vi "Event Handler.vi"(8 "error in (no error)":errorcluster, 10 "Stop Event Handler":refnum<user-event>, 11 "XYGraphOverview in":refnum<class "XYGraphOverview.lvclass">) -> (0 "error out":errorcluster)   [LabVIEW 2020, in "XYGraphOverview.lvlib" / "XYGraphOverview.lvclass"]
doc: "The <b>Event Handler VI</b> is a dynamic dispatch VI that should be overwritten if events are needed to create the enhanced QControl. \n\nBy inheriting from the main Control.lvclass the overwritten <b>Event Handler VI</b> will be launched asynchronously in the initialization of the QControl.\n<b> </b> <b> </b>\n©2016 Q Software Innovations, LLC (QSI)\nwritten by Quentin Alldredge\nproduced in LabVIEW 2015\n\nsupport@qsoftwareinnovations.com\nwww.qsoftwareinnovations.com\n\nAll rights reserved.\n\nRedistribution and use in source and binary forms, with or without modification, are permitted provided that the following conditions are met:\n\n * Redistributions of source code must retain the above copyright notice, this list of conditions and the following disclaimer.\n * Redistributions in binary form must reproduce the above copyright notice, this list of conditions and the following disclaimer in the documentation and/or other materials provided with the distribution.\n * Neither the name of Q Software Innovations, LLC. nor the names of its contributors may be used to endorse or promote products derived from this software without specific prior written permission.\n\nTHIS SOFTWARE IS PROVIDED BY THE COPYRIGHT HOLDERS AND CONTRIBUTORS \"AS IS\" AND ANY EXPRESS OR IMPLIED WARRANTIES, INCLUDING, BUT NOT LIMITED TO, THE IMPLIED WARRANTIES OF MERCHANTABILITY AND FITNESS FOR A PARTICULAR PURPOSE ARE DISCLAIMED. IN NO EVENT SHALL THE COPYRIGHT OWNER OR CONTRIBUTORS BE LIABLE FOR ANY DIRECT, INDIRECT, INCIDENTAL, SPECIAL, EXEMPLARY, OR CONSEQUENTIAL DAMAGES (INCLUDING, BUT NOT LIMITED TO, PROCUREMENT OF SUBSTITUTE GOODS OR SERVICES; LOSS OF USE, DATA, OR PROFITS; OR BUSINESS INTERRUPTION) HOWEVER CAUSED AND ON ANY THEORY OF LIABILITY, WHETHER IN CONTRACT, STRICT LIABILITY, OR TORT (INCLUDING NEGLIGENCE OR OTHERWISE) ARISING IN ANY WAY OUT OF THE USE OF THIS SOFTWARE, EVEN IF ADVISED OF THE POSSIBILITY OF SUCH DAMAGE."
uses:
  XYGraphOverview.lvclass
  XYGraphOverview.lvclass/XYGraphOverview.ctl
  X Range Change User Event Data.ctl
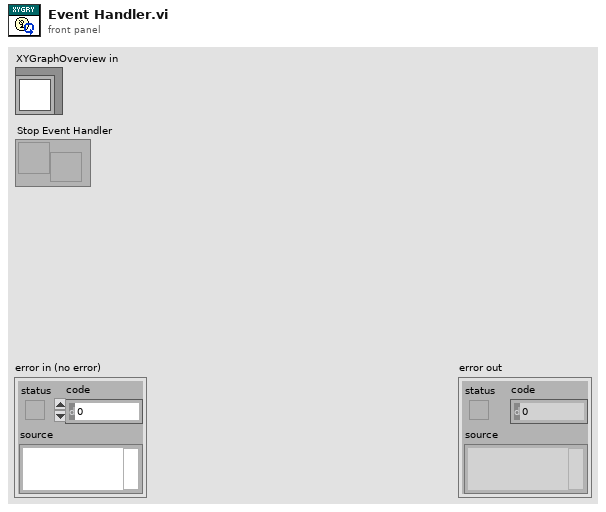
[diagram p1: front panel]
types:
  T1 = typedef "XYGraphOverview.lvlib/XYGraphOverview.lvclass/X Range Change User Event Data.ctl" = cluster{"Lower Range":dbl, "Upper Range":dbl, "All":bool}
  T2 = typedef "XYGraphOverview.lvlib/XYGraphOverview.lvclass/Command.ctl" = enum16{"Update Data", "Update Limit", "Zoom"}
  T3 = typedef "LVPoint32TypeDef.ctl" = cluster{"Horizontal":i32, "Vertical":i32}
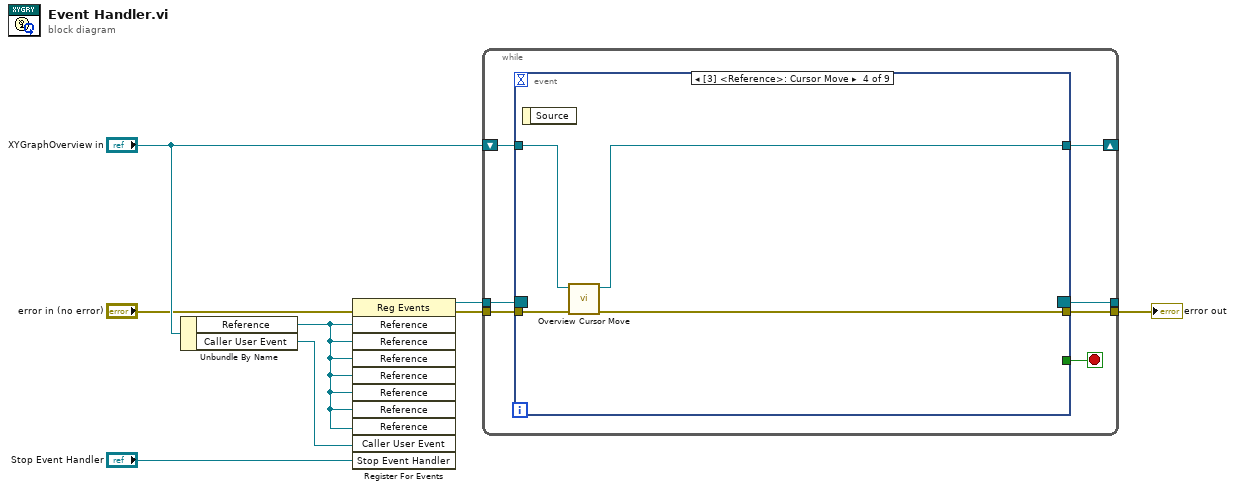
[diagram p0: block diagram]
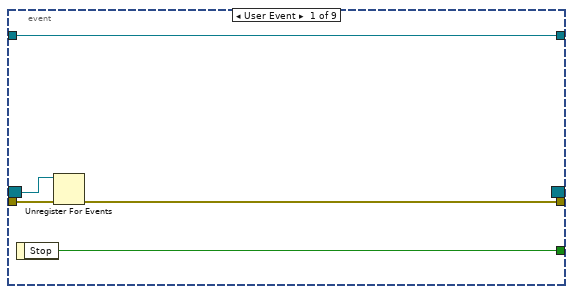
[diagram p2: hidden frame]
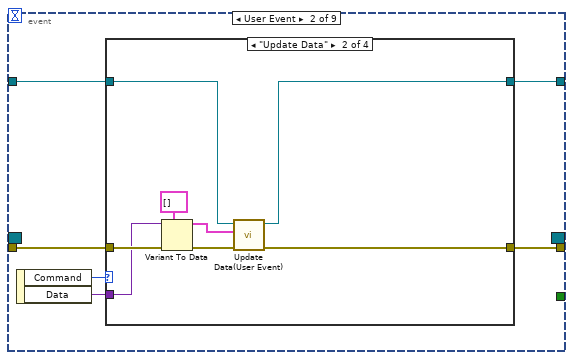
[diagram p3: hidden frame]
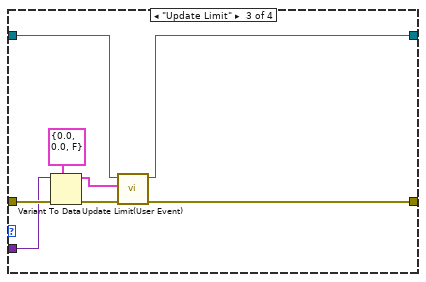
[diagram p5: hidden frame]
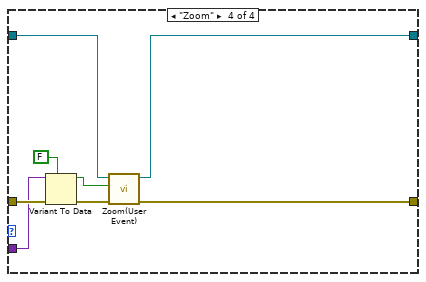
[diagram p6: hidden frame]
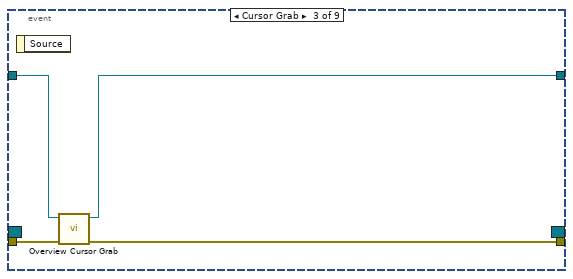
[diagram p7: hidden frame]
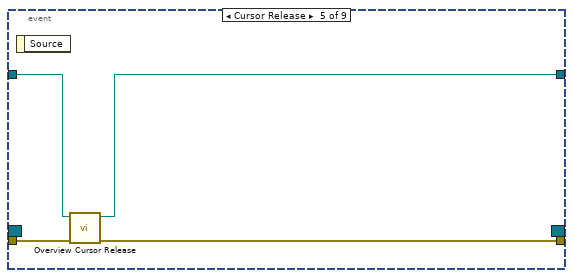
[diagram p8: hidden frame]
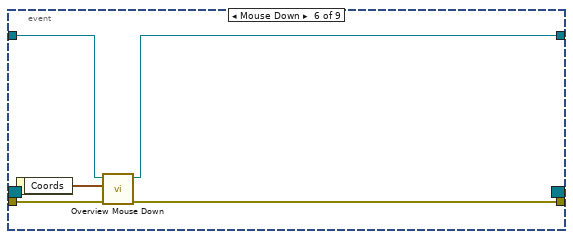
[diagram p9: hidden frame]
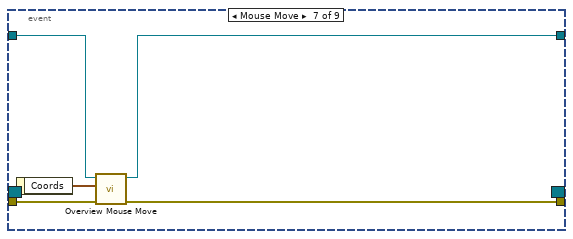
[diagram p10: hidden frame]
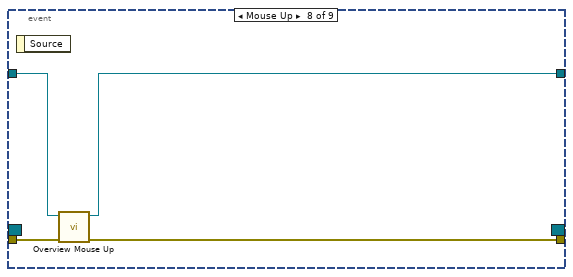
[diagram p11: hidden frame]
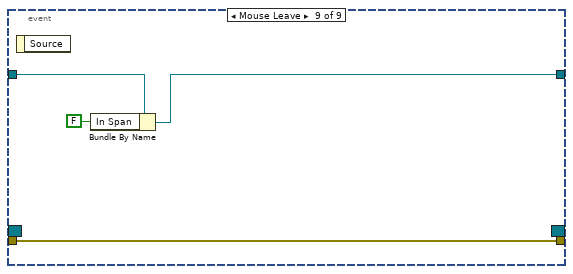
[diagram p12: hidden frame]
diagram:
  n1 = Unbundle By Name("XYGraphOverview in") -> ("Reference"=w4:refnum<vi>, "Caller User Event"=w3:refnum<user-event>)
  n2 = register-events(error in="error in (no error)", w4, w4, w4, w4, w4, w4, w4, w3, "Stop Event Handler") -> (reference out=w7:refnum<event-registration>, error out=w6:errorcluster)  [unwired: 1 in]
  n3 = while {
    tunnel: w7 -> [w15]
    tunnel: w6 -> [w13]
    tunnel: [w12] -> w1
    tunnel: [w10] -> _
    shift-right: [w9] -> _
    shift-left: "XYGraphOverview in" -> [w14]
    stop <- w11 stop-if-true
    n4 = event shown="[3] <Reference>: Cursor Move" {
      selector: w15 -> [w18 _ _ _ _ _ _ _ _]
      dyn-events: [_ _ _ _ _ _ _ _ _] -> w10
      timeout: _ -> [_ _ _ _ _ _ _ _ _]
      tunnel: w14 -> [w16 w25 w55 w59 w62 w68 w73 w76 w82]
      tunnel: w13 -> [w19 w24 w56 w60 w64 w69 w74 w78 w79]
      tunnel: [w17 w23 w53 w58 w63 w67 w71 w77 w79] -> w12
      tunnel: [w20 _ _ _ _ _ _ _ _] -> w11
      tunnel: [w16 w21 w54 w57 w61 w65 w70 w75 w80] -> w9
      event User Event {
        n5 = event-data() -> ("Stop"=w20:bool)  [unwired: 1 in]
        n6 = Unregister For Events(event registration refnum=w18, error in=w19) -> (error out=w17:errorcluster)
      }
      event User Event {
        n7 = event-data() -> ("Command"=w26:T2, "Data"=w22:variant)  [unwired: 1 in]
        n8 = case shown="\"Update Data\"" w26 {
          tunnel: w25 -> [w27 w31 w39 w51]
          tunnel: w24 -> [w28 w36 w44 w49]
          tunnel: [w28 w30 w37 w52] -> w23
          tunnel: w22 -> [_ w35 w43 w48]
          tunnel: [w27 w29 w38 w50] -> w21
          frame Default {
          }
          frame "Update Data" {
            n9 = Variant To Data(error in=w36, type=cluster{"X":dbl[], "Y":dbl[]}[] [] ("Data"), Variant=w35) -> (data=w32:cluster{"X":dbl[], "Y":dbl[]}[], error out=w33:errorcluster)
            n10 = call "Update Data(User Event).vi"("error in (no error)"=w33, "Data"=w32, "XYGraphOverview in"=w31) -> ("error out"=w30:errorcluster, "XYGraphOverview out"=w29:refnum<class "XYGraphOverview.lvclass">)  [unwired: 7 in]
          }
          frame "Update Limit" {
            n11 = Variant To Data(error in=w44, type=T1 {"Lower Range"=0.0, "Upper Range"=0.0, "All"=FALSE} ("X Range Change User Event Data"), Variant=w43) -> (data=w40:T1, error out=w41:errorcluster)
            n12 = call "Update Limit(User Event).vi"("error in (no error)"=w41, "X Range Change User Event Data"=w40, "XYGraphOverview in"=w39) -> ("error out"=w37:errorcluster, "XYGraphOverview out"=w38:refnum<class "XYGraphOverview.lvclass">)  [unwired: 7 in]
          }
          frame "Zoom" {
            n13 = Variant To Data(error in=w49, type=FALSE, Variant=w48) -> (data=w45:bool, error out=w46:errorcluster)
            n14 = call "Zoom(User Event).vi"("error in (no error)"=w46, "Zoom"=w45, "XYGraphOverview in"=w51) -> ("error out"=w52:errorcluster, "XYGraphOverview out"=w50:refnum<class "XYGraphOverview.lvclass">)  [unwired: 7 in]
          }
        }
      }
      event Cursor Grab {
        n15 = event-data() -> ()  [unwired: 1 in, 1 out]
        n16 = call "Overview Cursor Grab.vi"("error in (no error)"=w56, "XYGraphOverview in"=w55) -> ("error out"=w53:errorcluster, "XYGraphOverview out"=w54:refnum<class "XYGraphOverview.lvclass">)  [unwired: 8 in]
      }
      event Cursor Move {
        n17 = event-data() -> ()  [unwired: 1 in, 1 out]
        n18 = call "Overview Cursor Move.vi"("error in"=w60, "XYGraphOverview in"=w59) -> ("error out"=w58:errorcluster, "XYGraphOverview out"=w57:refnum<class "XYGraphOverview.lvclass">)  [unwired: 8 in]
      }
      event Cursor Release {
        n19 = event-data() -> ()  [unwired: 1 in, 1 out]
        n20 = call "Overview Cursor Release.vi"("error in"=w64, "XYGraphOverview in"=w62) -> ("error out"=w63:errorcluster, "XYGraphOverview out"=w61:refnum<class "XYGraphOverview.lvclass">)  [unwired: 8 in]
      }
      event Mouse Down {
        n21 = event-data() -> ("Coords"=w66:T3)  [unwired: 1 in]
        n22 = call "Overview Mouse Down.vi"("error in"=w69, "Coords"=w66, "XYGraphOverview in"=w68) -> ("error out"=w67:errorcluster, "XYGraphOverview out"=w65:refnum<class "XYGraphOverview.lvclass">)  [unwired: 7 in]
      }
      event Mouse Move {
        n23 = event-data() -> ("Coords"=w72:T3)  [unwired: 1 in]
        n24 = call "Overview Mouse Move.vi"("error in"=w74, "Coords"=w72, "XYGraphOverview in"=w73) -> ("error out"=w71:errorcluster, "XYGraphOverview out"=w70:refnum<class "XYGraphOverview.lvclass">)  [unwired: 7 in]
      }
      event Mouse Up {
        n25 = event-data() -> ()  [unwired: 1 in, 1 out]
        n26 = call "Overview Mouse Up.vi"("error in"=w78, "XYGraphOverview in"=w76) -> ("error out"=w77:errorcluster, "XYGraphOverview out"=w75:refnum<class "XYGraphOverview.lvclass">)  [unwired: 8 in]
      }
      event Mouse Leave {
        n27 = event-data() -> ()  [unwired: 1 in, 1 out]
        n28 = Bundle By Name(cluster=w82, "In Span"=FALSE) -> (w80:refnum<class "XYGraphOverview.lvclass">)
      }
    }
  }
  "error out" <- w1
